vi "RT_NetStream_ESP.vi"(8 "error in (no error)":errorcluster, 10 "output cluster":T1={"N_chan"=0, "Input Rate (Hz)"=0.0, "Acq Time (s)"=0.0, "NumOfWarmupIters"=0, "Size fifo"=0, "Period NCL (ms)"=0, "Timeout fifo Read"=0, "Size Sent Array"=0, "Output offsets"=[], "Input offsets"=[0.0, 0.0, 0.0, 0.0, 0.0, 0.0, 0.0, 0.0]}, 11 "rt fifo":refnum<k33>) -> (3 "error out 3":errorcluster)   [LabVIEW 2021]
uses:
  parametersRT.ctl
panel:
  out "Array":dbl[][](array[numeric])
  in  "Stream":bool
  out "output array":sgl[][](array[numeric])
  out "Waveform Chart 2":sgl[][](graph)
  out "Waveform Chart":sgl[](graph)
  out "Stream on?":string
  out "element out":dbl[](array[numeric])
  out "Numeric":i32
  out "i":dbl
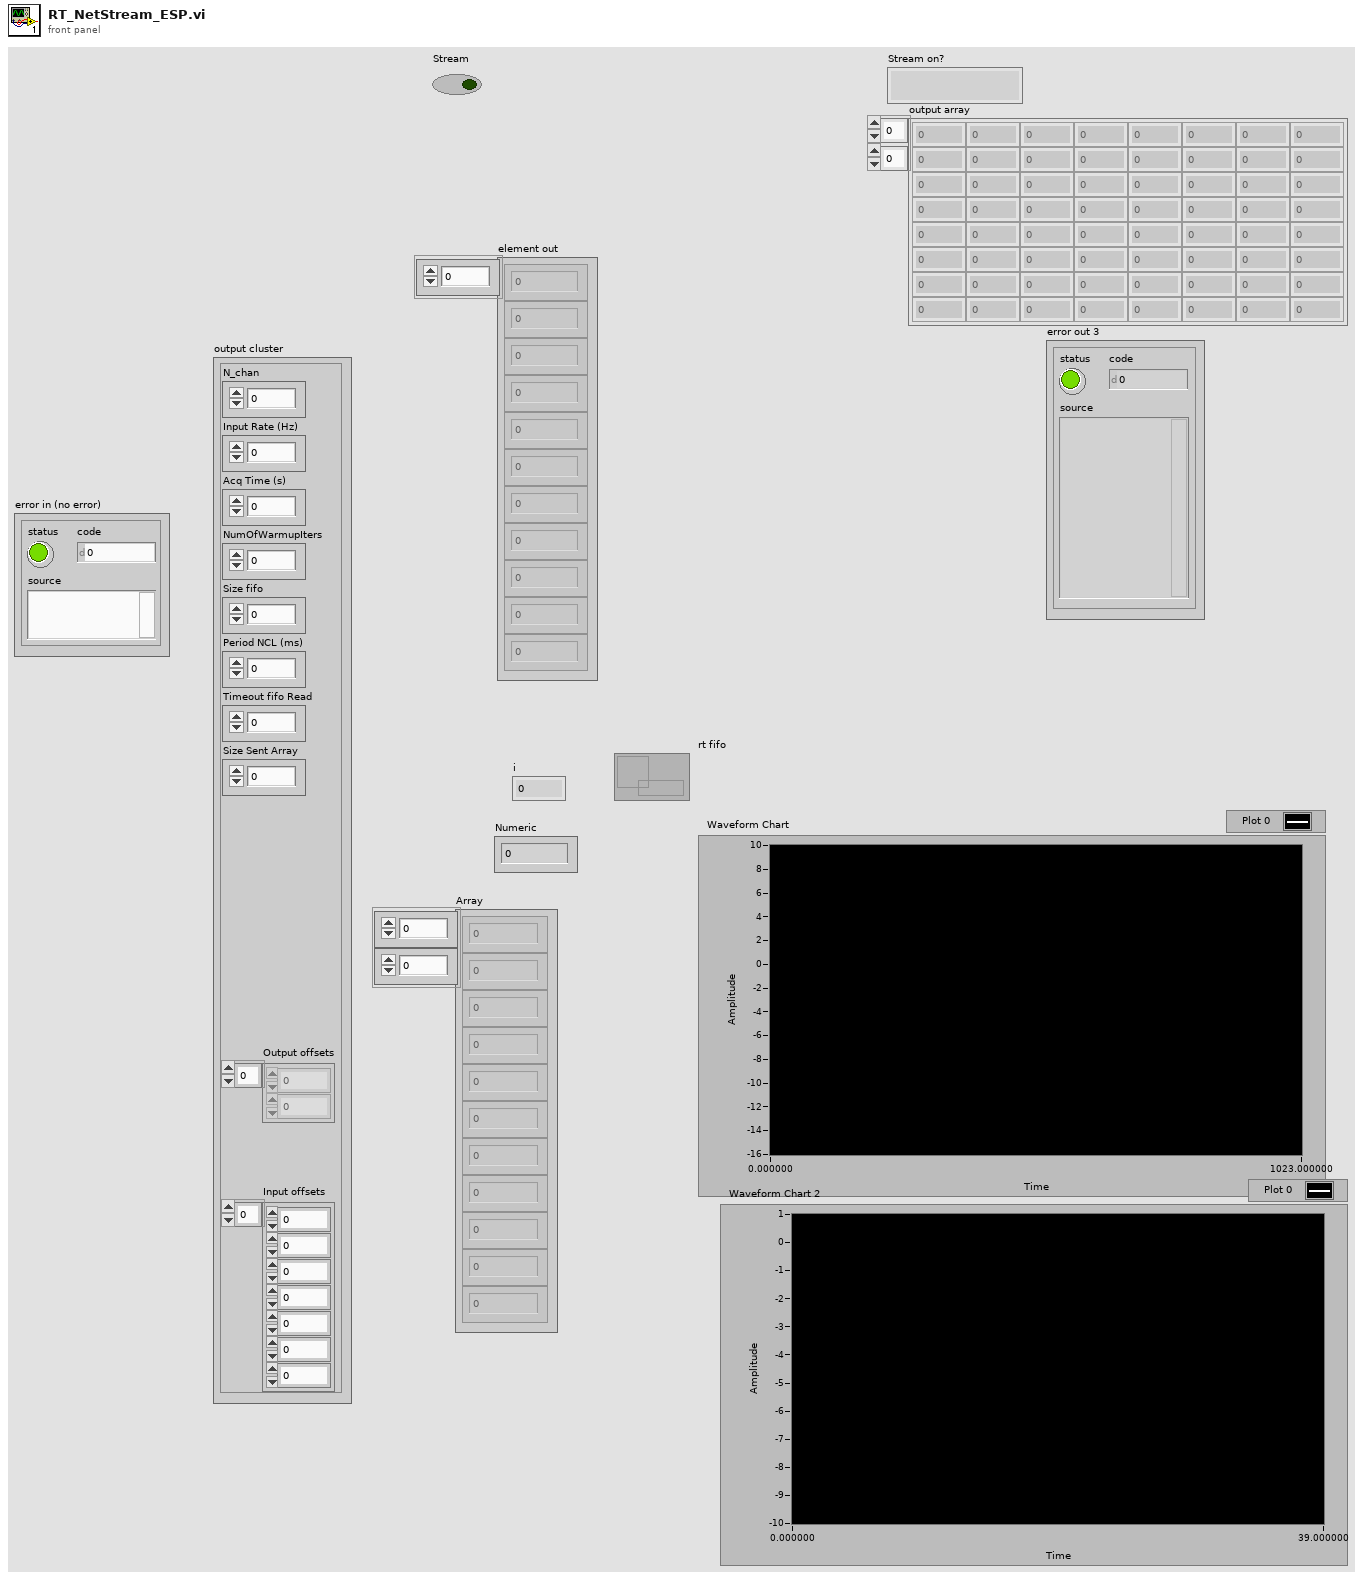
[diagram p1: front panel]
types:
  T1 = typedef "parametersRT.ctl" = cluster{"N_chan":u32, "Input Rate (Hz)":dbl, "Acq Time (s)":dbl, "NumOfWarmupIters":u32, "Size fifo":u32, "Period NCL (ms)":i64, "Timeout fifo Read":i32, "Size Sent Array":i32, "Output offsets":dbl[], "Input offsets":dbl[]}
  T2 = enum16{"Standard", "Buffered", "CRLF", "Immediate"}
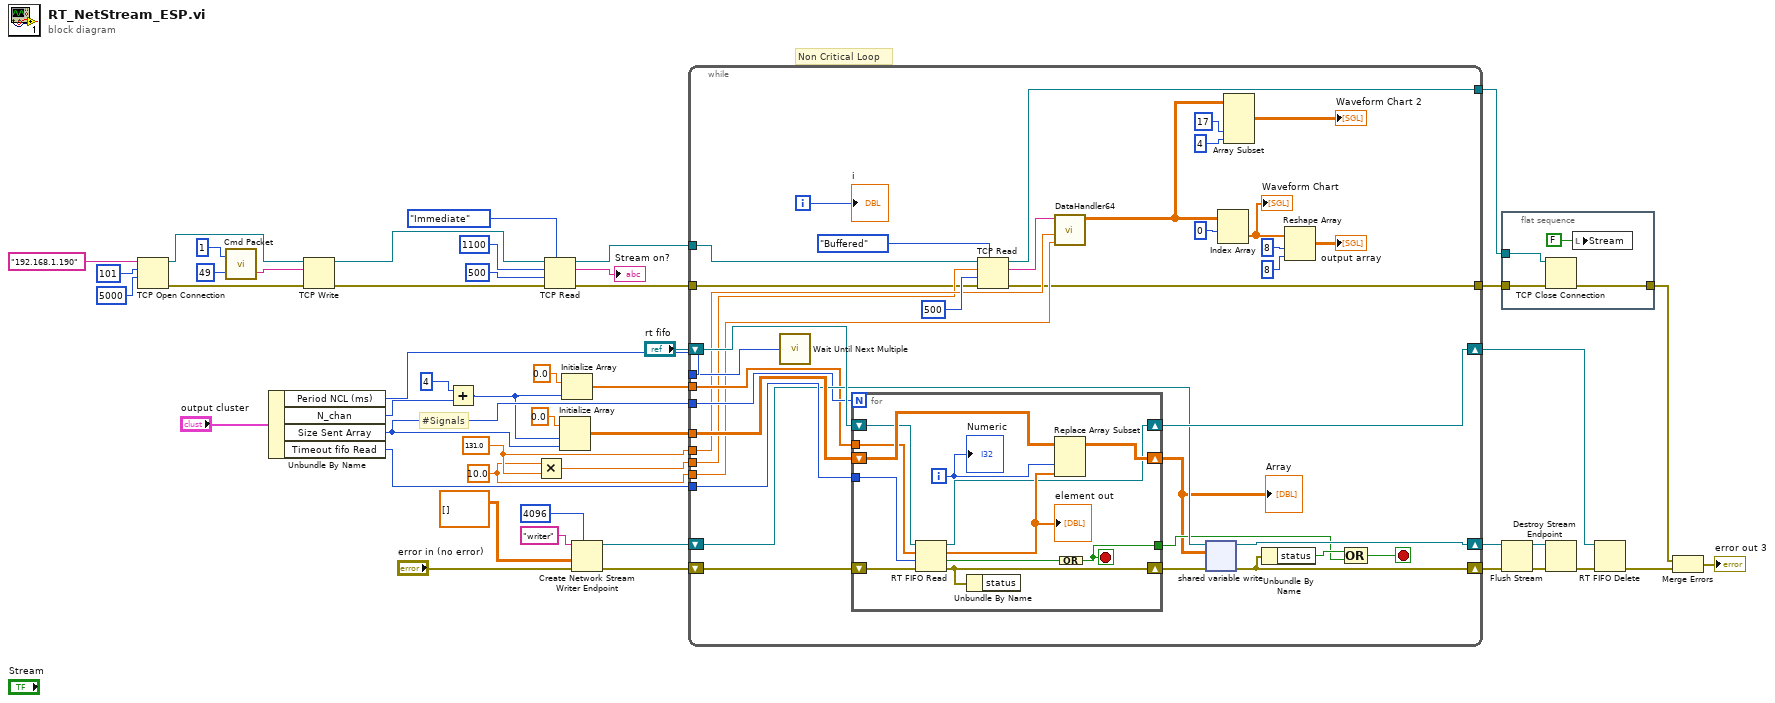
[diagram p0: block diagram]
diagram:
  w10 = 10.0 ("Sampling Rate")
  w11 = 131.0 ("y")
  # "#Signals"
  # "Non Critical Loop"
  n1 = TCP Open Connection(address="192.168.1.190", remote port or service name=u16 101 ("Port"), timeout ms (60000)=5000) -> (connection ID=w22:refnum<k5>, error out=w14:errorcluster)  [unwired: 2 in]
  n2 = call "Cmd Packet.vi"("Command Byte"=49 ("data in"), "Parameter Byte"=1 ("data in")) -> ("Command Packet Byte String"=w25:string)  [unwired: 1 out]
  n3 = Unbundle By Name("output cluster") -> ("Period NCL (ms)"=w32:i64, "N_chan"=w31:u32, "Size Sent Array"=w30:i32, "Timeout fifo Read"=w29:i32)
  n4 = TCP Write(connection ID=w22, data in=w25, error in (no error)=w14) -> (connection ID out=w23:refnum<k5>, error out=w13:errorcluster)  [unwired: 1 in, 1 out]
  n5 = Add(x=4, y=w31) -> (x+y=w1:u32)
  n6 = Multiply(x=w10, y=w11) -> (x*y=w9:dbl)
  n7 = TCP Read(connection ID=w23, bytes to read=1100, error in (no error)=w13, 7:T2."Immediate" ("mode (standard)"), 9:500 ("timeout ms (25000)")) -> (connection ID out=w8:refnum<k5>, data out=→"Stream on?":string, error out=w7:errorcluster)
  n8 = Initialize Array(0.0 ("element"), w1, w30) -> (w46:dbl[][])
  n9 = Initialize Array(0.0 ("element"), w1) -> (w33:dbl[])
  n10 = Create Network Stream Writer Endpoint(7:4096 ("writer buffer size"), 8:"error in (no error)", 9:dbl[][] [], 11:"writer" ("writer name")) -> (0:w26:errorcluster, 3:w34:refnum<k21>)  [unwired: 3 in]
  n11 = while {
    tunnel: w46 -> [w82]
    tunnel: w30 -> [w74]
    shift-right: [w70] -> w42
    shift-left: w26 -> [w81]
    tunnel: w29 -> [w80]
    shift-right: [w78] -> w39
    shift-left: "rt fifo" -> [w79]
    shift-right: [w77] -> w40
    shift-left: w34 -> [w75]
    tunnel: w33 -> [w73]
    tunnel: w32 -> [w72]
    tunnel: w11 -> [w55]
    tunnel: w10 -> [w53]
    tunnel: w9 -> [w54]
    tunnel: w8 -> [w52]
    tunnel: w7 -> [w51]
    tunnel: [w50] -> w6
    tunnel: [w49] -> w5
    i -> [w69]
    stop <- w84 stop-if-true
    n12 = call "Wait Until Next Multiple"("Count(mSec)"=w72) -> ()  [unwired: 1 out]
    n13 = for {
      N: w74 -> [_]
      shift-right: [w96] -> w68
      shift-left: w82 -> [w95]
      shift-right: [w87] -> w76
      shift-left: w81 -> [w92]
      tunnel: w80 -> [w91]
      shift-right: [w89] -> w78
      shift-left: w79 -> [w90]
      tunnel: w73 -> [w88]
      tunnel: [w85] -> w71
      i -> [w93]
      stop <- w85 stop-if-true
      n14 = RT FIFO Read(0:w90, 1:w88, 2:w91, 3:w92) -> (8:w89:refnum<k33>, 9:w94:dbl[], 10:w86:bool, 11:w87:errorcluster)  [unwired: 1 out]
      "element out" <- w94
      n15 = Unbundle By Name(w87) -> ()  [unwired: 1 out]
      n16 = Replace Array Subset(array=w95, new element=w94, index (col)=w93) -> (w96:dbl[][])  [unwired: 1 in]
      n17 = Compound Arithmetic op=OR(w86) -> (w85:bool)
      "Numeric" <- w93
    }
    "Array" <- w68
    n18 = TCP Read(connection ID=w52, bytes to read=w54, error in (no error)=w51, 7:T2."Buffered" ("mode (standard)"), 9:500 ("timeout ms (25000)")) -> (connection ID out=w49:refnum<k5>, data out=w67:string, error out=w50:errorcluster)
    n19 = call "DataHandler64.vi"("Data Cycles Per Buffer"=w53, "Rx Packet Byte size"=w55, "data out"=w67) -> ("Data"=w56:sgl[][])  [unwired: 2 in, 4 out]
    n20 = shared-variable-write(w75, w76, w68) -> (w77:refnum<k21>, w70:errorcluster)  [unwired: 1 in, 1 out]
    n21 = Index Array(array=w56, index (row)=0 ("Channel")) -> (element=w58:sgl[])  [unwired: 1 in]
    "Waveform Chart" <- w58
    n22 = Array Subset(array=w56, index (col)=17 ("index"), length (col)=4 ("length")) -> (→"Waveform Chart 2":sgl[][])  [unwired: 2 in]
    n23 = Unbundle By Name(w70) -> ("status"=w83:bool)
    n24 = Reshape Array(w58, 8 ("dimension size"), 8 ("dimension size")) -> (→"output array":sgl[][])
    n25 = Compound Arithmetic op=OR(w83, w71) -> (w84:bool)
    "i" <- w69
  }
  n26 = flat-sequence {
    tunnel: w6 -> [w99]
    tunnel: [w98] -> w3
    tunnel: w5 -> [w97]
    frame #0 {
      n27 = TCP Close Connection(connection ID=w97, error in (no error)=w99) -> (error out=w98:errorcluster)  [unwired: 1 in, 1 out]
      n28 = local write "Stream"(FALSE) -> ()
    }
  }
  n29 = Flush Stream(8:w42, 11:w40) -> (0:w41:errorcluster, 3:w43:refnum<k21>)  [unwired: 2 in, 1 out]
  n30 = Destroy Stream Endpoint(8:w41, 11:w43) -> (0:w38:errorcluster)
  n31 = RT FIFO Delete(0:w39, 3:w38) -> (11:w2:errorcluster)  [unwired: 1 in]
  n32 = Merge Errors(w3, w2) -> (→"error out 3":errorcluster)
